vi "navX_SPI_CRC.vi"(0 "Message":u8[](array[numeric])=[255, 43, 176, 52, 27, 0, 240]) -> (1 "Message with CRC":u8[](array[numeric]), 2 "CRC":u8 format="%.0x")   [LabVIEW 2019]
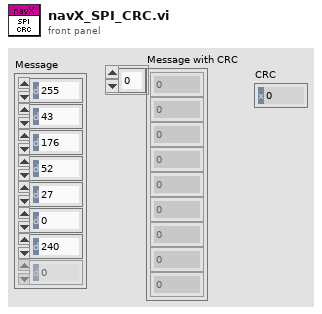
[diagram p1: front panel]
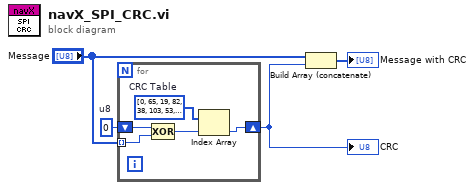
[diagram p0: block diagram]
diagram:
  w3 = u8 0  # u8
  n1 = for {
    shift-right: [w5] -> w1
    shift-left: w3 -> [w9]
    tunnel: "Message" -> [w8] mode=indexing
    w7 = i32[] [0, 65, 19, 82, 38, 103, 53, 116, 76, 13, 95, 30, 106, 43, 121, 56, 9, 72, 26, 91, 47, 110, 60, 125, 69, 4, 86, 23, 99, 34, 112, 49, 18, 83, 1, 64, 52, 117, 39, 102, 94, 31, 77, 12, 120, 57, 107, 42, 27, 90, 8, 73, 61, 124, 46, 111, 87, 22, 68, 5, 113, 48, 98, 35, 36, 101, 55, 118, 2, 67, 17, 80, 104, 41, 123, 58, 78, 15, 93, 28, 45, 108, 62, 127, 11, 74, 24, 89, 97, 32, 114, 51, 71, 6, 84, 21, 54, 119, 37, 100, 16, 81, 3, 66, 122, 59, 105, 40, 92, 29, 79, 14, 63, 126, 44, 109, 25, 88, 10, 75, 115, 50, 96, 33, 85, 20, 70, 7, 72, 9, 91, 26, 110, 47, 125, 60, 4, 69, 23, 86, 34, 99, 49, 112, 65, 0, 82, 19, 103, 38, 116, 53, 13, 76, 30, 95, 43, 106, 56, 121, 90, 27, 73, 8, 124, 61, 111, 46, 22, 87, 5, 68, 48, 113, 35, 98, 83, 18, 64, 1, 117, 52, 102, 39, 31, 94, 12, 77, 57, 120, 42, 107, 108, 45, 127, 62, 74, 11, 89, 24, 32, 97, 51, 114, 6, 71, 21, 84, 101, 36, 118, 55, 67, 2, 80, 17, 41, 104, 58, 123, 15, 78, 28, 93, 126, 63, 109, 44, 88, 25, 75, 10, 50, 115, 33, 96, 20, 85, 7, 70, 119, 54, 100, 37, 81, 16, 66, 3, 59, 122, 40, 105, 29, 92, 14, 79]  # CRC Table
    n2 = Compound Arithmetic op=XOR(w9, w8) -> (w6:i32)
    n3 = Index Array(array=w7, index=w6) -> (element=w5:i32)
  }
  "CRC" <- w1
  n4 = Build Array (concatenate)("Message", w1) -> (→"Message with CRC":i32[])
